vi "Event - 1000 msec.vi"() -> ()   [LabVIEW 2011]
doc: "This VI calls a FGV Timer and resets the timer every 1000 msec. The purpose is to demonstrate using multiple instances of an object in a LabVIEW application. The FGV is designed for only one instance and cannot be used in this use case.\n\nAAL 9/09"
panel:
  out "Elapsed Time (ms)":u32
  in  "Exit":bool
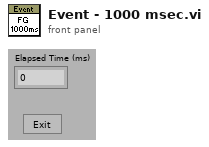
[diagram p1: front panel]
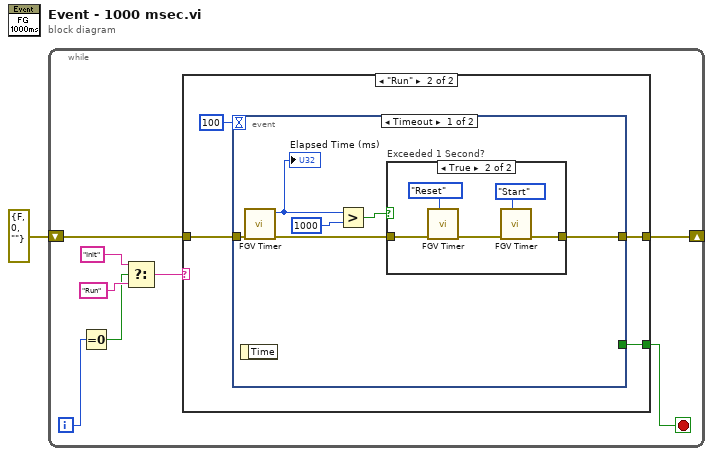
[diagram p0: block diagram]
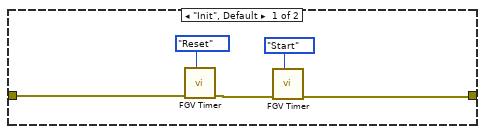
[diagram p2: hidden frame]
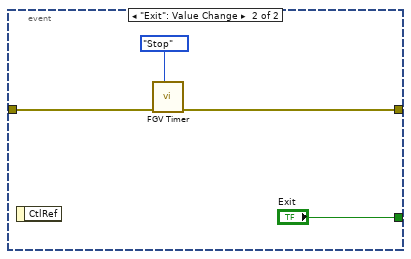
[diagram p4: hidden frame]
diagram:
  n1 = while {
    shift-right: [w3] -> _
    shift-left: errorcluster {"status"=FALSE, "code"=0, "source"=""} ("error out") -> [w2]
    i -> [w8]
    stop <- w9 stop-if-true
    n2 = Equal To 0?(x=w8) -> (x = 0?=w6:bool)
    n3 = Select(t="Init", s=w6, f="Run") -> (s? t:f=w4:string)
    n4 = case shown="\"Run\"" w4 {
      tunnel: [_ w17] -> w9
      tunnel: [w12 w16] -> w3
      tunnel: w2 -> [w14 w15]
      frame "Init", Default {
        n5 = call "FGV Timer.vi"("Method (Get Time)"=enum16{"Start", "Stop", "Reset", "Get Time"}."Reset", "error in (no error)"=w14) -> ("error out"=w13:errorcluster)  [unwired: 7 in, 2 out]
        n6 = call "FGV Timer.vi"("Method (Get Time)"=enum16{"Start", "Stop", "Reset", "Get Time"}."Start", "error in (no error)"=w13) -> ("error out"=w12:errorcluster)  [unwired: 7 in, 2 out]
      }
      frame "Run" {
        n7 = event shown="[0] Timeout" {
          selector: _ -> [_ _]
          dyn-events: _ -> [_ _]
          timeout: 100 -> [_ _]
          tunnel: [_ "Exit"] -> w17
          tunnel: [w20 w31] -> w16
          tunnel: w15 -> [w19 w32]
          event Timeout {
            n8 = event-data() -> ()  [unwired: 1 in, 1 out]
            n9 = call "FGV Timer.vi"("error in (no error)"=w19) -> ("error out"=w21:errorcluster, "Elapsed Time (ms)"=w22:u32)  [unwired: 8 in, 1 out]
            "Elapsed Time (ms)" <- w22
            n10 = Greater?(x=w22, y=u32 1000) -> (0:w23:bool)
            n11 = case "Exceeded 1 Second?" shown="True" w23 {
              tunnel: w21 -> [w25 w28]
              tunnel: [w25 w26] -> w20
              frame False {
              }
              frame True {
                n12 = call "FGV Timer.vi"("Method (Get Time)"=enum16{"Start", "Stop", "Reset", "Get Time"}."Reset", "error in (no error)"=w28) -> ("error out"=w27:errorcluster)  [unwired: 7 in, 2 out]
                n13 = call "FGV Timer.vi"("Method (Get Time)"=enum16{"Start", "Stop", "Reset", "Get Time"}."Start", "error in (no error)"=w27) -> ("error out"=w26:errorcluster)  [unwired: 7 in, 2 out]
              }
            }
          }
          event "Exit": Value Change {
            n14 = event-data() -> ()  [unwired: 1 in, 1 out]
            n15 = call "FGV Timer.vi"("Method (Get Time)"=enum16{"Start", "Stop", "Reset", "Get Time"}."Stop", "error in (no error)"=w32) -> ("error out"=w31:errorcluster)  [unwired: 7 in, 2 out]
          }
        }
      }
    }
  }
